vi "DrawTopMenuRectangle.vi"(7 "Collection in":refnum<class "Collection.lvclass">, 8 "error in (no error)":errorcluster, 11 "Menu in":refnum<class "Menu.lvclass">) -> (0 "error out":errorcluster, 3 "Menu out":refnum<class "Menu.lvclass">, 5 "Collection out":refnum<class "Collection.lvclass">)   [LabVIEW 2021, in "Menu.lvlib" / "Menu.lvclass"]
uses:
  Menu.lvclass
  Menu.lvclass/Menu.ctl
  Picture2D/src/Rectangle/Rectangle.lvclass
  Picture2D/src/Collection/Collection.lvclass
  Picture2D/src/Point/Point.lvclass
  C:/GitHub/Picture2D/src/Polygone/Polygone.lvclass
  C:/GitHub/Picture2D/src/Shape/Shape.lvclass
  C:/GitHub/Picture2D/src/Picture2D/Picture2D.lvclass
  C:/GitHub/Picture2D/src/IDrawable/IDrawable.lvclass
  C:/GitHub/Picture2D/src/IMovable/IMovable.lvclass
  C:/GitHub/Picture2D/src/IRotatable/IRotatable.lvclass
  C:/GitHub/Picture2D/src/IScalable/IScalable.lvclass
  C:/GitHub/Picture2D/src/Rectangle/Rectangle.lvclass
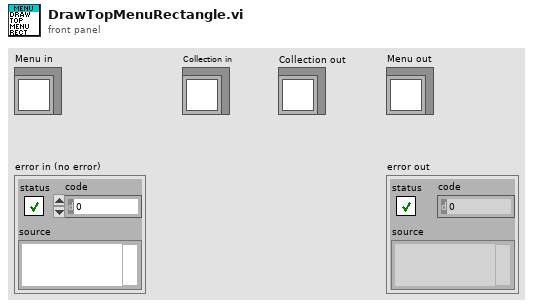
[diagram p1: front panel]
types:
  T1 = typedef "LVBoundsTypeDef.ctl" = cluster{"Width":u32, "Height":u32}
  T2 = typedef "Menu.lvlib/Menu.lvclass/MenuColors.ctl" = cluster{"Text":refnum<class "Color.lvclass">, "HiliteText":refnum<class "Color.lvclass">, "Background":refnum<class "Color.lvclass">, "BorderColor":refnum<class "Color.lvclass">, "Hilite":refnum<class "Color.lvclass">}
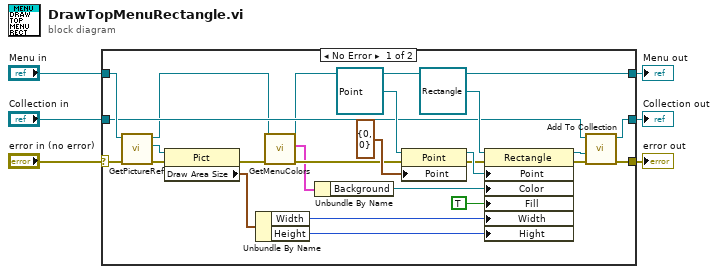
[diagram p0: block diagram]
diagram:
  n1 = case shown="No Error" "error in (no error)" {
    selector: "error in (no error)" -> [w23 w33]
    tunnel: [w13 w33] -> w5
    tunnel: [w9 w32] -> w3
    tunnel: "Menu in" -> [w22 w32]
    tunnel: "Collection in" -> [w17 w31]
    tunnel: [w16 w31] -> w1
    frame No Error {
      n2 = call "GetPictureRef.vi"("error in (no error)"=w23, "Menu in"=w22) -> ("error out"=w14:errorcluster, "PictRef"=w20:refnum<vi>, "Menu out"=w10:refnum<class "Menu.lvclass">)  [unwired: 7 in]
      n3 = property on="Property Node" class="Pict"(reference=w20, error in=w14) -> (error out=w12:errorcluster, "Draw Area Size"=w21:T1)  [unwired: 1 out]
      n4 = Unbundle By Name(w21) -> ("Width"=w19:u32, "Height"=w18:u32)
      n5 = call "GetMenuColors.vi"("error in (no error)"=w12, "Menu in"=w10) -> ("error out"=w11:errorcluster, "MenuColors"=w8:T2, "Menu out"=w9:refnum<class "Menu.lvclass">)  [unwired: 7 in]
      n6 = Unbundle By Name(w8) -> ("Background"=w7:refnum<class "Color.lvclass">)
      n7 = property class="Point"(reference=refnum<class "Point.lvclass"> refnum, error in=w11, "Point"=cluster{"x":i16, "y":i16} {"x"=0, "y"=0} ("Point:All Elements")) -> (reference out=w28:refnum<class "Point.lvclass">, error out=w15:errorcluster)
      n8 = property class="Rectangle"(reference=refnum<class "Rectangle.lvclass"> refnum ("Picture2D.lvlib:Rectangle"), error in=w15, "Point"=w28, "Color"=w7, "Fill"=TRUE, "Width"=w19, "Hight"=w18) -> (reference out=w30:refnum<class "Rectangle.lvclass">, error out=w24:errorcluster)
      n9 = call-dynamic "Add To Collection.vi"("error in (no error)"=w24, "IDrawable"=w30, "Collection in"=w17) -> ("error out"=w13:errorcluster, "Collection out"=w16:refnum<class "Collection.lvclass">)  [unwired: 7 in]
    }
    frame Error {
    }
  }
  "error out" <- w5
  "Menu out" <- w3
  "Collection out" <- w1
